vi "Wrap Position.vi"(10 "Position":refnum<class "Vector 2D.lvclass">, 11 "Camera in":refnum<class "Camera.lvclass">) -> (3 "Wrapped Position":refnum<class "Vector 2D.lvclass">)   [LabVIEW 2021, in "Camera.lvclass"]
uses:
  Camera.lvclass
  Re-use Libraries/Vector 2D/Vector 2D.lvclass
  Camera.lvclass/Camera.ctl
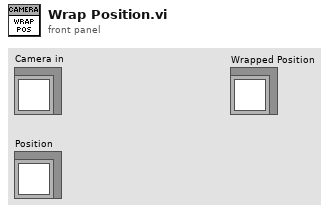
[diagram p1: front panel]
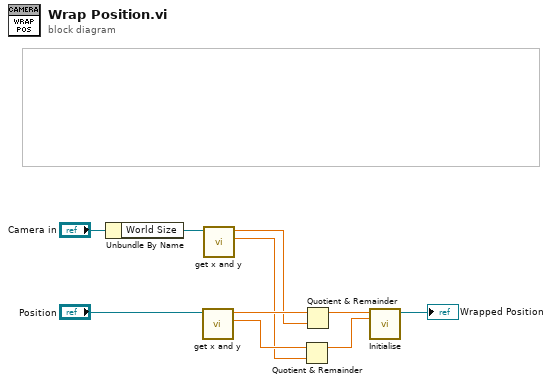
[diagram p0: block diagram]
diagram:
  n1 = Unbundle By Name("Camera in") -> ("World Size"=w9:refnum<class "Vector 2D.lvclass">)
  n2 = call "get x and y.vi"("Vector 2D in"="Position") -> ("y"=w5:sgl, "x"=w7:sgl)  [unwired: 9 in]
  n3 = call "get x and y.vi"("Vector 2D in"=w9) -> ("y"=w4:sgl, "x"=w6:sgl)  [unwired: 9 in]
  n4 = Quotient & Remainder(x=w5, y=w4) -> (x-y*floor(x/y)=w2:sgl)  [unwired: 1 out]
  n5 = Quotient & Remainder(x=w7, y=w6) -> (x-y*floor(x/y)=w3:sgl)  [unwired: 1 out]
  n6 = call "Initialise.vi"("y"=w2, "x"=w3) -> ("Vector 2D out"=→"Wrapped Position":refnum<class "Vector 2D.lvclass">)  [unwired: 9 in]
